vi "Init.vi"(9 "Dt":dbl, 10 "Size":i32, 11 "DFT-1 in":refnum<class "DFT1.lvclass">) -> (3 "DFT-1 out":refnum<class "DFT1.lvclass">)   [LabVIEW 2014, in "Exponential Fit Library.lvlib" / "DFT1.lvclass"]
doc: "Calculate the sine and cosine of the angular frequency (wk = 2*pi*k/(N*dt)) ."
uses:
  DFT1.lvclass
  DFT1.lvclass/DFT1.ctl
  Fit Exponential.lvclass
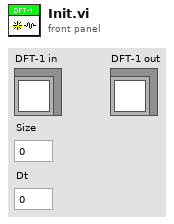
[diagram p1: front panel]
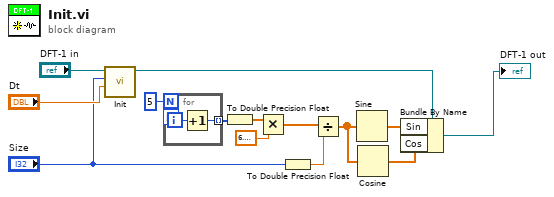
[diagram p0: block diagram]
diagram:
  n1 = call-parent "Init.vi"("Dt"="Dt", "Size"="Size", "Fit Exponential in"="DFT-1 in") -> ("Fit Exponential out"=w4:refnum<class "DFT1.lvclass">)  [unwired: 8 in]
  n2 = for {
    N: 5 -> [_]
    tunnel: [w15] -> w8 mode=indexing
    workers-P: _ -> [_]
    i -> [w16]
    n3 = Increment(x=w16) -> (x+1=w15:i32)
  }
  n4 = To Double Precision Float(number=w8) -> (double precision float=w9:dbl[])
  n5 = Multiply(x=w9, y=6.283185307179586) -> (x*y=w6:dbl[])
  n6 = To Double Precision Float(number="Size") -> (double precision float=w11:dbl)
  n7 = Divide(x=w6, y=w11) -> (x/y=w12:dbl[])
  n8 = Sine(x=w12) -> (sin(x)=w3:dbl[])
  n9 = Cosine(x=w12) -> (cos(x)=w2:dbl[])
  n10 = Bundle By Name(cluster=w4, "Sin"=w3, "Cos"=w2) -> (→"DFT-1 out":refnum<class "DFT1.lvclass">)
